vi "rename_document.vi"(0 "Device In":T1, 1 "Name":string, 5 "did":string, 11 "error in":errorcluster) -> (4 "Device Out":T1, 15 "error out":errorcluster)   [LabVIEW 2019]
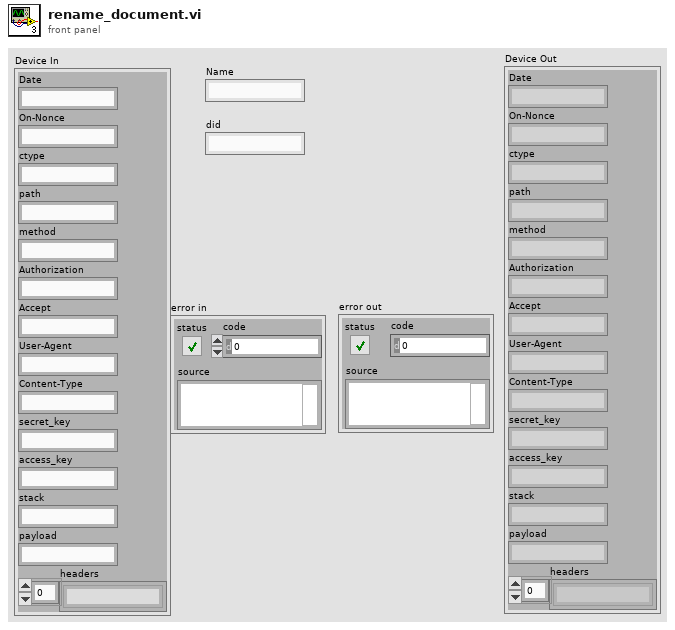
[diagram p1: front panel]
types:
  T1 = cluster{"Date":string, "On-Nonce":string, "ctype":string, "path":string, "method":string, "Authorization":string, "Accept":string, "User-Agent":string, "Content-Type":string, "secret_key":string, "access_key":string, "stack":string, "payload":string, "headers":string[]}
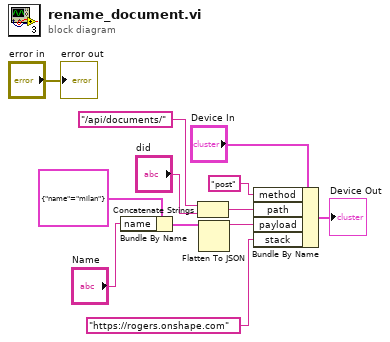
[diagram p0: block diagram]
diagram:
  n1 = Bundle By Name(cluster=cluster{"name":string} {"name"="milan"}, "name"="Name") -> (w9:cluster{"name":string})
  n2 = Concatenate Strings("/api/documents/" ("payload"), "did") -> (w4:string)
  n3 = Flatten To JSON(anything=w9) -> (JSON string=w3:string)  [unwired: 2 in, 1 out]
  n4 = Bundle By Name(cluster="Device In", "method"="post" ("Method"), "path"=w4, "payload"=w3, "stack"="https://rogers.onshape.com" ("stacks")) -> (→"Device Out":T1)
  "error out" <- "error in"
